vi "StahlPS_Pbus.Read_DB.vi"(0 "i ref in":refnum<vi>, 5 "error in (no error)":errorcluster) -> (14 "i ref out":refnum<vi>, 19 "error out (no error)":errorcluster)   [LabVIEW 2014, in "StahlPS_Pbus.lvlib"]
doc: "This VI reads outall important Values from the Database (or directly from the Baseprocess Class)"
uses:
  StahlPS_Pbus.lvlib
  CSCore/BaseProcess/BaseProcess.lvlib
  CSCore/CSSystem/CoreLib/CoreLib.lvlib
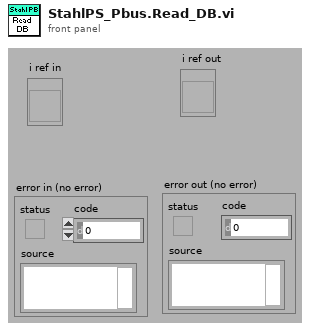
[diagram p1: front panel]
types:
  T1 = typedef "BaseProcess.lvlib/BaseProcess.i attribute.ctl" = cluster{"EventStatus":string, "EventError":i32, "PresetEvtWatchD":i32, "PresetPdcWatchD":i32, "EventTimeout":i32, "PeriodicInterval":i32, "Interface":string[], "Address":string[], "Special":string[], "PeriodicError":i32, "PeriodicStatus":string, "SuperProc":string, "Descriptors":T2[], "CaseRef":refnum<vi>, "PdcRef":refnum<vi>, "Thread Ref":refnum<vi>, "eventErrorID":i32, "eventStatusID":i32, "periodicErrorID":i32, "periodicStatusID":i32, "pdcCtrID":i32}
  T2 = typedef "BaseProcess.lvlib/BaseProcess.descriptor definition.ctl" = cluster{"selector":string, "descriptor":T3}
  T3 = typedef "BaseProcess.lvlib/BaseProcess.descriptor string definition.ctl" = string
  T4 = typedef "StahlPS_Pbus.lvlib/StahlPS_Pbus.i attribute.ctl" = cluster{"Type":string, "CALC_FACTOR_SET_VOLTAGE":dbl, "CALC_FACTOR_GET_VOLTAGE":dbl, "CALC_FACTOR_GET_CURRENT":dbl, "CALC_FACTOR_SET_CURRENT ":dbl, "REG_VALUE":dbl, "Sign":bool, "setVoltIDs":i32[], "Elektrode Names":string[]}
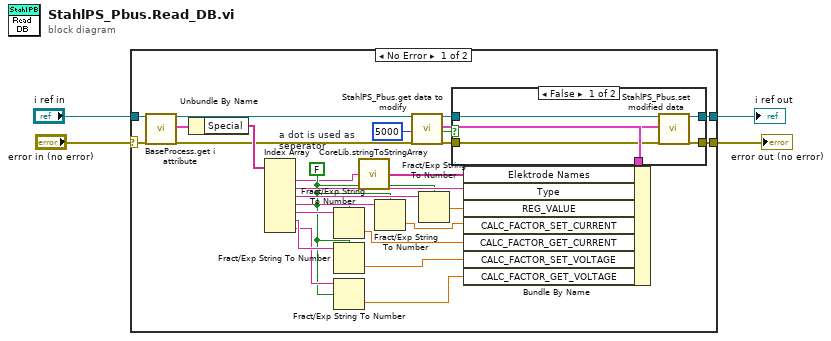
[diagram p0: block diagram]
diagram:
  n1 = case shown="No Error" "error in (no error)" {
    selector: "error in (no error)" -> [w28 w41]
    tunnel: [w31 w41] -> w1
    tunnel: "i ref in" -> [w30 w40]
    tunnel: [w32 w40] -> w3
    frame No Error {
      w9 = FALSE  # a dot is used as seperator
      n2 = call "BaseProcess.get i attribute.vi"("i ref in"=w30, "error in (no error)"=w28) -> ("i ref out"=w29:refnum<vi>, "i attribute"=w21:T1, "error out"=w17:errorcluster)  [unwired: 15 in]
      n3 = Unbundle By Name(w21) -> ("Special"=w20:string[])
      n4 = Index Array(array=w20) -> (element #1=w6:string, element #2=w16:string, element #3=w15:string, element #4=w14:string, element #5=w13:string, element #6=w12:string, element #7=w10:string)  [unwired: 7 in]
      n5 = Fract/Exp String To Number(use system decimal point (T)=w9, string=w13) -> (number=w23:dbl)  [unwired: 2 in, 1 out]
      n6 = Fract/Exp String To Number(use system decimal point (T)=w9, string=w12) -> (number=w11:dbl)  [unwired: 2 in, 1 out]
      n7 = Fract/Exp String To Number(use system decimal point (T)=w9, string=w10) -> (number=w22:dbl)  [unwired: 2 in, 1 out]
      n8 = call "CoreLib.stringToStringArray.vi"("String"=w6) -> ("Array"=w5:string[])
      n9 = Fract/Exp String To Number(use system decimal point (T)=w9, string=w14) -> (number=w24:dbl)  [unwired: 2 in, 1 out]
      n10 = call "StahlPS_Pbus.get data to modify.vi"("i ref in"=w29, "ms timeout (10000)"=5000, "error in (no error)"=w17) -> ("i ref out"=w27:refnum<vi>, "i attribute"=w19:T4, "timed out"=w8:bool, "error out"=w26:errorcluster)  [unwired: 13 in]
      n11 = Fract/Exp String To Number(use system decimal point (T)=w9, string=w15) -> (number=w25:dbl)  [unwired: 2 in, 1 out]
      n12 = Bundle By Name(cluster=w19, "Elektrode Names"=w5, "Type"=w16, "REG_VALUE"=w25, "CALC_FACTOR_SET_CURRENT"=w24, "CALC_FACTOR_GET_CURRENT"=w23, "CALC_FACTOR_SET_VOLTAGE"=w11, "CALC_FACTOR_GET_VOLTAGE"=w22) -> (w18:T4)
      n13 = case shown="False" w8 {
        tunnel: [w37 w39] -> w32
        tunnel: [w36 w38] -> w31
        tunnel: w27 -> [w35 w39]
        tunnel: w26 -> [w34 w38]
        tunnel: w18 -> [w33 _]
        frame False {
          n14 = call "StahlPS_Pbus.set modified data.vi"("i ref in"=w35, "i attribute"=w33, "error in (no error)"=w34) -> ("i ref out"=w37:refnum<vi>, "error out"=w36:errorcluster)  [unwired: 15 in]
        }
        frame True {
        }
      }
    }
    frame Error {
    }
  }
  "error out (no error)" <- w1
  "i ref out" <- w3
